vi "display_1s_stim_9s_ISI_CS1_CS2_blocks_no_trigger3.vi"() -> ()   [LabVIEW 2019]
uses:
  <vilib>/Analysis/Matrix/Datatypes/RealMatrix.ctl
  <vilib>/Utility/file.llb/Write Delimited Spreadsheet (DBL).vi
  <vilib>/Analysis/Matrix/NI_Matrix.lvlib
panel:
  out "ISI Time":dbl
  out "Stim TS":dbl
  out "Output":dbl[][](array[numeric])
  out "Output frame":T1
  out "Array temp1":T1
  out "Elapsed Time":dbl
  out "Display":bool=TRUE
  out "Trial":u32=1
  out "reward":dbl[](array[numeric])
  out "stim_id":dbl[](array[numeric])
  out "stim_loaded":dbl
  out "Timings":dbl[](array[numeric])
  out "Stimuli Loaded?":bool
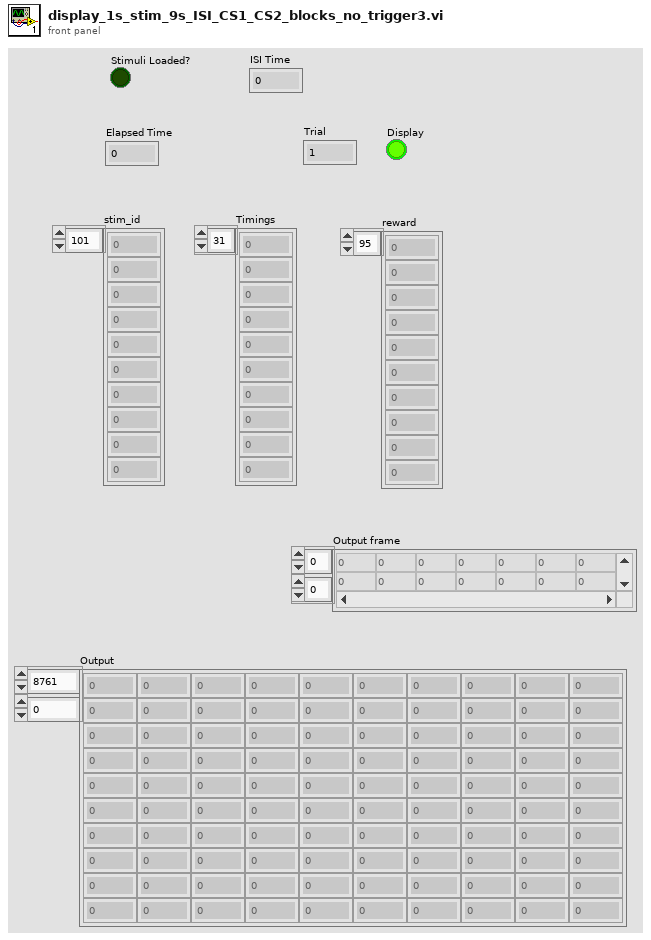
[diagram p1: front panel]
types:
  T1 = typedef "NI_Matrix.lvlib/RealMatrix.ctl" = dbl[][]
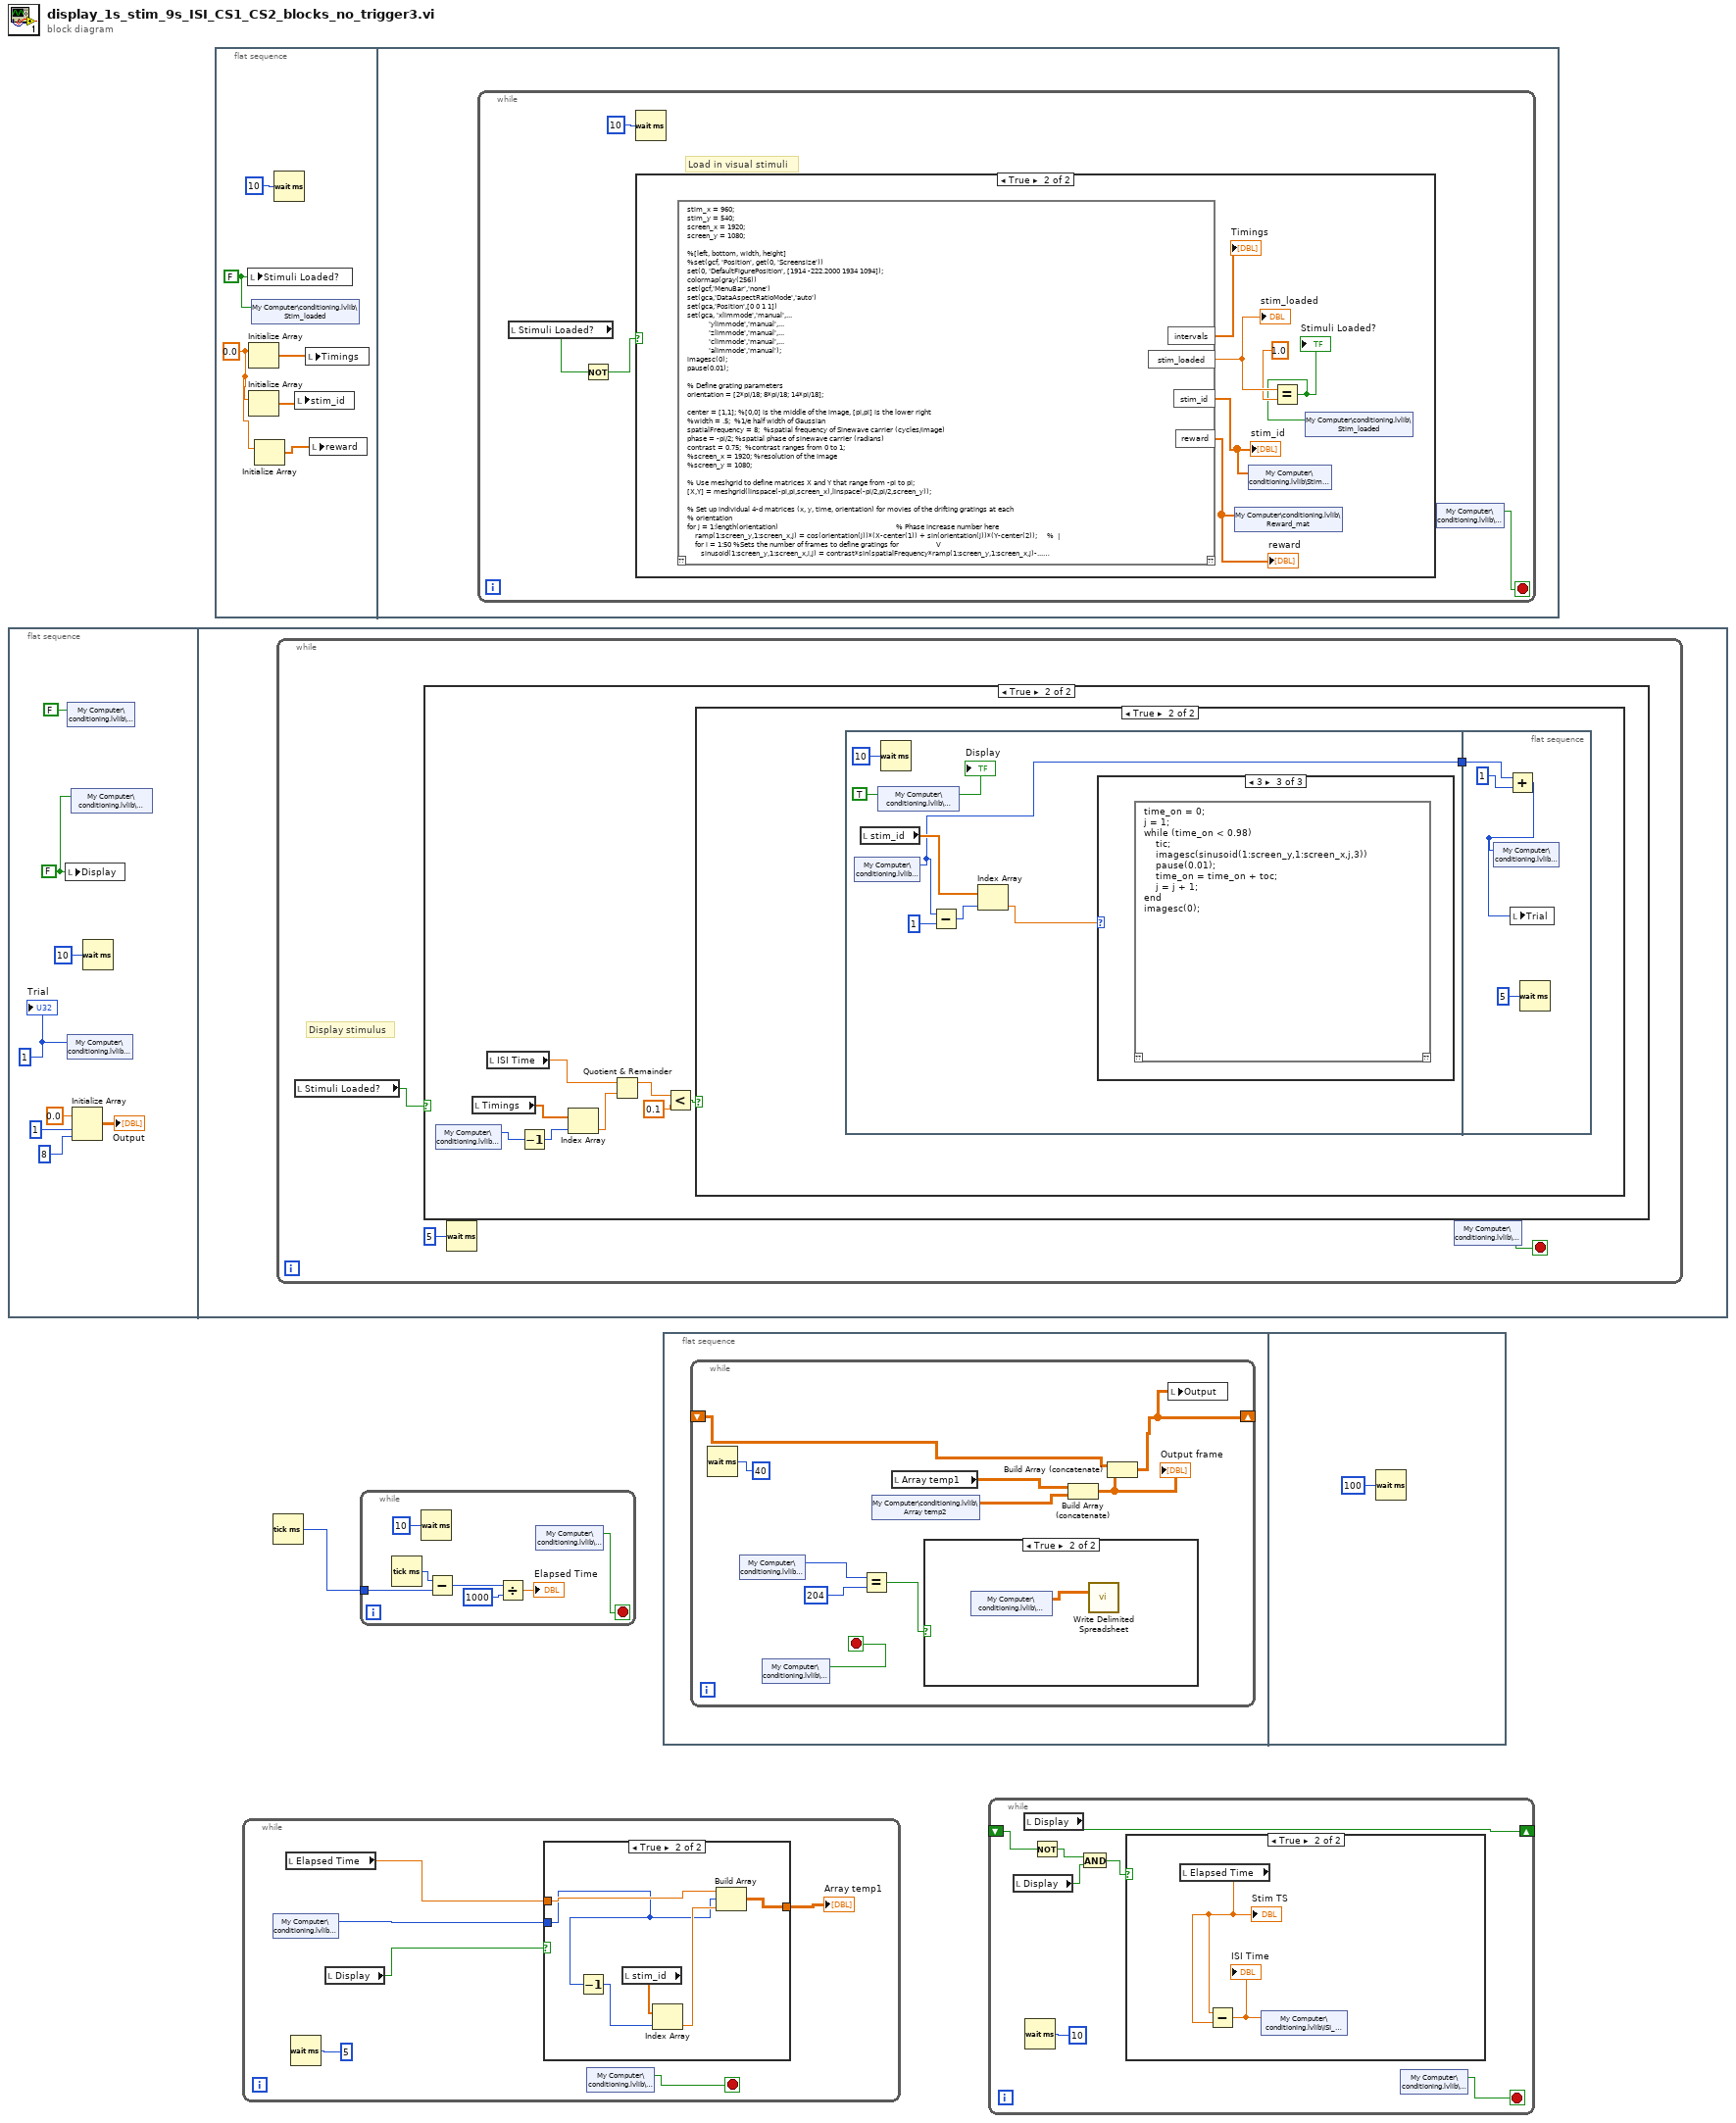
[diagram p0: block diagram]
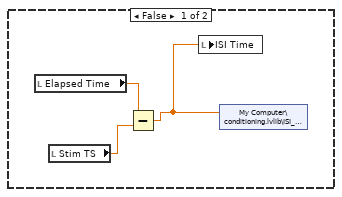
[diagram p2: hidden frame]
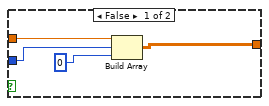
[diagram p3: hidden frame]
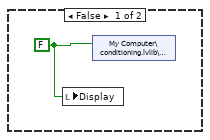
[diagram p7: hidden frame]
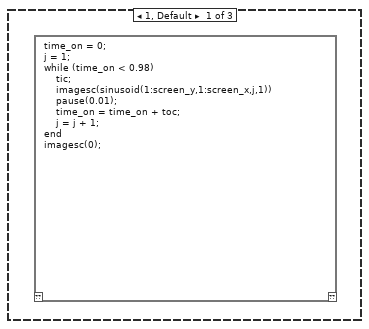
[diagram p8: hidden frame]
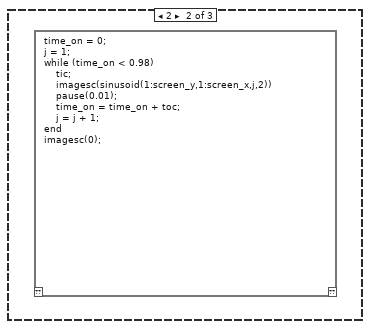
[diagram p9: hidden frame]
diagram:
  n1 = flat-sequence {
    frame #0 {
      w7 = FALSE ("Display")
      w9 = u32 1 ("Trial")
      n2 = local write "Display"(w7) -> ()
      n3 = shared-variable "My Computer\\conditioning.lvlib\\Stop"(FALSE ("Stop")) -> ()  [unwired: 1 in, 1 out]
      n4 = shared-variable "My Computer\\conditioning.lvlib\\Trial"(w9) -> ()  [unwired: 1 in, 1 out]
      n5 = shared-variable "My Computer\\conditioning.lvlib\\Display"(w7) -> ()  [unwired: 1 in, 1 out]
      n6 = Initialize Array(0.0 ("element"), 1 ("dimension size"), 8 ("dimension size")) -> (→"Output":dbl[][])
      n7 = Wait (ms)(milliseconds to wait=u32 10) -> ()  [unwired: 1 out]
      "Trial" <- w9
    }
    frame #1 {
      n8 = while {
        stop <- w11 stop-if-true
        # "Display stimulus"
        n9 = local read "Stimuli Loaded?"() -> (w10:bool)
        n10 = case shown="True" w10 {
          frame False {
          }
          frame True {
            n11 = shared-variable "My Computer\\conditioning.lvlib\\Trial"() -> (w16:u32)  [unwired: 1 in, 1 out]
            n12 = local read "Timings"() -> (w17:dbl[])
            n13 = local read "ISI Time"() -> (w13:dbl)
            n14 = Decrement(x=w16) -> (x-1=w15:u32)
            n15 = Index Array(array=w17, index=w15) -> (element=w14:dbl)
            n16 = Quotient & Remainder(x=w13, y=w14) -> (x-y*floor(x/y)=w20:dbl)  [unwired: 1 out]
            n17 = Less?(x=w20, y=0.1) -> (x < y?=w18:bool)
            n18 = case shown="True" w18 {
              frame False {
                w21 = FALSE ("Display")
                n19 = local write "Display"(w21) -> ()
                n20 = shared-variable "My Computer\\conditioning.lvlib\\Display"(w21) -> ()  [unwired: 1 in, 1 out]
              }
              frame True {
                n21 = flat-sequence {
                  tunnel: [w25] -> w22
                  tunnel: w22 -> [w33]
                  frame #0 {
                    w27 = TRUE ("Boolean")
                    n22 = shared-variable "My Computer\\conditioning.lvlib\\Trial"() -> (w25:u32)  [unwired: 1 in, 1 out]
                    n23 = local read "stim_id"() -> (w28:dbl[])
                    n24 = shared-variable "My Computer\\conditioning.lvlib\\Display"(w27) -> ()  [unwired: 1 in, 1 out]
                    n25 = Wait (ms)(milliseconds to wait=u32 10) -> ()  [unwired: 1 out]
                    n26 = Subtract(x=w25, y=u32 1) -> (x-y=w26:u32)
                    n27 = Index Array(array=w28, index=w26) -> (element=w23:dbl)
                    n28 = case shown="3" w23 {
                      frame 1, Default {
                        n29 = script code="time_on = 0;\nj = 1;\nwhile (time_on < 0.98)\n    tic;\n    imagesc(sinusoid(1:screen_y,1:screen_x,j,1))\n    pause(0.01);\n    time_on = time_on + toc;\n    j = j + 1;\nend\nimagesc(0);"() -> ()  [unwired: 1 in, 1 out]
                      }
                      frame 2 {
                        n30 = script code="time_on = 0;\nj = 1;\nwhile (time_on < 0.98)\n    tic;\n    imagesc(sinusoid(1:screen_y,1:screen_x,j,2))\n    pause(0.01);\n    time_on = time_on + toc;\n    j = j + 1;\nend\nimagesc(0);"() -> ()  [unwired: 1 in, 1 out]
                      }
                      frame 3 {
                        n31 = script code="time_on = 0;\nj = 1;\nwhile (time_on < 0.98)\n    tic;\n    imagesc(sinusoid(1:screen_y,1:screen_x,j,3))\n    pause(0.01);\n    time_on = time_on + toc;\n    j = j + 1;\nend\nimagesc(0);"() -> ()  [unwired: 1 in, 1 out]
                      }
                    }
                    "Display" <- w27
                  }
                  frame #1 {
                    n32 = Add(x=w33, y=u32 1) -> (x+y=w31:u32)
                    n33 = shared-variable "My Computer\\conditioning.lvlib\\Trial"(w31) -> ()  [unwired: 1 in, 1 out]
                    n34 = local write "Trial"(w31) -> ()
                    n35 = Wait (ms)(milliseconds to wait=u32 5) -> ()  [unwired: 1 out]
                  }
                }
              }
            }
          }
        }
        n36 = Wait (ms)(milliseconds to wait=u32 5) -> ()  [unwired: 1 out]
        n37 = shared-variable "My Computer\\conditioning.lvlib\\Stop"() -> (w11:bool)  [unwired: 1 in, 1 out]
      }
    }
  }
  n38 = flat-sequence {
    frame #0 {
      w36 = 0.0 ("element")
      w34 = FALSE ("Stimuli Loaded?")
      n39 = local write "Stimuli Loaded?"(w34) -> ()
      n40 = Initialize Array(w36) -> (w38:dbl[])  [unwired: 1 in]
      n41 = Initialize Array(w36) -> (w37:dbl[])  [unwired: 1 in]
      n42 = shared-variable "My Computer\\conditioning.lvlib\\Stim_loaded"(w34) -> ()  [unwired: 1 in, 1 out]
      n43 = Initialize Array(w36) -> (w35:dbl[])  [unwired: 1 in]
      n44 = Wait (ms)(milliseconds to wait=u32 10) -> ()  [unwired: 1 out]
      n45 = local write "stim_id"(w37) -> ()
      n46 = local write "Timings"(w38) -> ()
      n47 = local write "reward"(w35) -> ()
    }
    frame #1 {
      n48 = while {
        stop <- w42 stop-if-true
        # "Load in visual stimuli"
        n49 = local read "Stimuli Loaded?"() -> (w41:bool)
        n50 = Not(x=w41) -> (.not. x?=w40:bool)
        n51 = Wait (ms)(milliseconds to wait=u32 10) -> ()  [unwired: 1 out]
        n52 = case shown="True" w40 {
          frame False {
          }
          frame True {
            n53 = script code="stim_x = 960;\nstim_y = 540;\nscreen_x = 1920;\nscreen_y = 1080;\n\n%[left, bottom, width, height]\n%set(gcf, 'Position', get(0, 'Screensize'))\nset(0, 'DefaultFigurePosition', [1914 -222.2000 1934 1094]);\ncolormap(gray(256))\nset(gcf,'MenuBar','none')\nset(gca,'DataAspectRatioMode','auto')\nset(gca,'Position',[0 0 1 1])\nset(gca, 'xlimmode','manual',...\n           'ylimmode','manual',...\n           'zlimmode','manual',...\n           'climmode','manual',...\n           'alimmode','manual');\nimagesc(0);\npause(0.01);\n\n% Define grating parameters\norientation = [2*pi/18; 8*pi/18; 14*pi/18];\n\ncenter = [1,1]; %[0,0] is the middle of the image, [pi,pi] is the lower right\n%width = .5;  %1/e half width of Gaussian\nspatialFrequency = 8;  %spatial frequency of Sinewave carrier (cycles/image)\nphase = -pi/2; %spatial phase of sinewave carrier (radians)\ncontrast = 0.75;  %contrast ranges from 0 to 1;\n%screen_x = 1920; %resolution of the image  \n%screen_y = 1080;\n\n% Use meshgrid to define matrices X and Y that range from -pi to pi;\n[X,Y] = meshgrid(linspace(-pi,pi,screen_x),linspace(-pi/2,pi/2,screen_y));\n\n% Set up individual 4-d matrices (x, y, time, orientation) for movies of the drifting gratings at each\n% orientation\nfor j = 1:length(orientation)                                                            % Phase increase number here\n    ramp(1:screen_y,1:screen_x,j) = cos(orientation(j))*(X-center(1)) + sin(orientation(j))*(Y-center(2));     %  |\n    for i = 1:50 %Sets the number of frames to define gratings for                   V\n       sinusoid(1:screen_y,1:screen_x,i,j) = contrast*sin(spatialFrequency*ramp(1:screen_y,1:screen_x,j)-...\n           (phase+(2*pi*(i-1)*(-30)/360))); %Number before '/360' sets the phase increase\n    end\nend\n\nintervals = [ones(1,41)*10 ones(1,41)*11 ones(1,41)*12 ones(1,41)*13 ones(1,40)*14];\nintervals = intervals(randperm(204));\nstim_id = [ones(1,34)*3 ones(1,34)*1 ones(1,34)*2 ones(1,34)*3 ones(1,34)*1 ones(1,34)*2];\nreward = [ones(1,34)*0 ones(1,34)*1 ones(1,34)*1 ones(1,34)*0 ones(1,34)*1 ones(1,34)*1];\n\nstim_loaded = 1;" ("Script Node")() -> ("stim_loaded"=w49:dbl, "intervals"=→"Timings":dbl[], "stim_id"=w44:dbl[], "reward"=w46:dbl[])  [unwired: 1 in, 1 out]
            "stim_loaded" <- w49
            "stim_id" <- w44
            "reward" <- w46
            n54 = shared-variable "My Computer\\conditioning.lvlib\\Reward_mat"(w46) -> ()  [unwired: 1 in, 1 out]
            n55 = shared-variable "My Computer\\conditioning.lvlib\\Stim_ID"(w44) -> ()  [unwired: 1 in, 1 out]
            n56 = Equal?(x=w49, y=1.0) -> (x = y?=w45:bool)
            "Stimuli Loaded?" <- w45
            n57 = shared-variable "My Computer\\conditioning.lvlib\\Stim_loaded"(w45) -> ()  [unwired: 1 in, 1 out]
          }
        }
        n58 = shared-variable "My Computer\\conditioning.lvlib\\Stop"() -> (w42:bool)  [unwired: 1 in, 1 out]
      }
    }
  }
  n59 = while {
    stop <- w50 stop-if-true
    n60 = shared-variable "My Computer\\conditioning.lvlib\\Trial"() -> (w52:u32)  [unwired: 1 in, 1 out]
    n61 = local read "Elapsed Time"() -> (w54:dbl)
    n62 = Wait (ms)(milliseconds to wait=u32 5) -> ()  [unwired: 1 out]
    n63 = local read "Display"() -> (w51:bool)
    n64 = case shown="True" w51 {
      tunnel: w52 -> [w58 w61]
      tunnel: w54 -> [w59 w63]
      tunnel: [w57 w64] -> w53
      frame False {
        n65 = Build Array(w59, w58, u32 0 ("milliseconds to wait")) -> (w57:T1)
      }
      frame True {
        n66 = Decrement(x=w61) -> (x-1=w60:u32)
        n67 = local read "stim_id"() -> (w65:dbl[])
        n68 = Index Array(array=w65, index=w60) -> (element=w62:dbl)
        n69 = Build Array(w63, w61, w62) -> (w64:T1)
      }
    }
    "Array temp1" <- w53
    n70 = shared-variable "My Computer\\conditioning.lvlib\\Stop"() -> (w50:bool)  [unwired: 1 in, 1 out]
  }
  n71 = Tick Count (ms)() -> (millisecond timer value=w1:u32)
  n72 = while {
    tunnel: w1 -> [w69]
    stop <- w66 stop-if-true
    n73 = Tick Count (ms)() -> (millisecond timer value=w70:u32)
    n74 = Wait (ms)(milliseconds to wait=u32 10) -> ()  [unwired: 1 out]
    n75 = Subtract(x=w70, y=w69) -> (x-y=w67:u32)
    n76 = Divide(x=w67, y=u32 1000) -> (x/y=→"Elapsed Time":dbl)
    n77 = shared-variable "My Computer\\conditioning.lvlib\\Stop"() -> (w66:bool)  [unwired: 1 in, 1 out]
  }
  n78 = flat-sequence {
    frame #0 {
      n79 = while {
        shift-right: [w79] -> _
        shift-left: _ -> [w80]
        stop <- w82 stop-if-true
        n80 = Wait (ms)(milliseconds to wait=u32 40) -> ()  [unwired: 1 out]
        n81 = shared-variable "My Computer\\conditioning.lvlib\\Trial"() -> (w75:u32)  [unwired: 1 in, 1 out]
        n82 = shared-variable "My Computer\\conditioning.lvlib\\Stop"() -> (w82:bool)  [unwired: 1 in, 1 out]
        n83 = Equal?(x=w75, y=u32 204) -> (x = y?=w73:bool)
        n84 = shared-variable "My Computer\\conditioning.lvlib\\Array temp2"() -> (w77:dbl[][])  [unwired: 1 in, 1 out]
        n85 = local read "Array temp1"() -> (w78:T1)
        n86 = case shown="True" w73 {
          frame False {
          }
          frame True {
            n87 = shared-variable "My Computer\\conditioning.lvlib\\Output"() -> (w83:dbl[][])  [unwired: 1 in, 1 out]
            n88 = call-poly <vilib>:"Write Delimited Spreadsheet.vi"("2D data"=w83) -> ()  [unwired: 13 in, 2 out]
          }
        }
        n89 = Build Array (concatenate)(w78, w77) -> (w76:T1)
        "Output frame" <- w76
        n90 = Build Array (concatenate) ("Build Matrix")(w80, w76) -> (w79:T1)
        n91 = local write "Output"(w79) -> ()
      }
    }
    frame #1 {
      n92 = Wait (ms)(milliseconds to wait=u32 100) -> ()  [unwired: 1 out]
    }
  }
  n93 = while {
    shift-right: [w89] -> _
    shift-left: _ -> [w88]
    stop <- w91 stop-if-true
    n94 = local read "Display"() -> (w86:bool)
    n95 = local read "Display"() -> (w89:bool)
    n96 = Wait (ms)(milliseconds to wait=u32 10) -> ()  [unwired: 1 out]
    n97 = Not(x=w88) -> (.not. x?=w87:bool)
    n98 = And(x=w87, y=w86) -> (x .and. y?=w85:bool)
    n99 = case shown="True" w85 {
      frame False {
        n100 = local read "Elapsed Time"() -> (w92:dbl)
        n101 = local read "Stim TS"() -> (w94:dbl)
        n102 = Subtract(x=w92, y=w94) -> (x-y=w93:dbl)
        n103 = local write "ISI Time"(w93) -> ()
        n104 = shared-variable "My Computer\\conditioning.lvlib\\ISI_Time"(w93) -> ()  [unwired: 1 in, 1 out]
      }
      frame True {
        n105 = local read "Elapsed Time"() -> (w95:dbl)
        "Stim TS" <- w95
        n106 = Subtract(x=w95, y=w95) -> (x-y=w96:dbl)
        "ISI Time" <- w96
        n107 = shared-variable "My Computer\\conditioning.lvlib\\ISI_Time"(w96) -> ()  [unwired: 1 in, 1 out]
      }
    }
    n108 = shared-variable "My Computer\\conditioning.lvlib\\Stop"() -> (w91:bool)  [unwired: 1 in, 1 out]
  }
